vi "speed.vi"(11 "rmp":dbl) -> (3 "km/h":dbl)   [LabVIEW 2016]
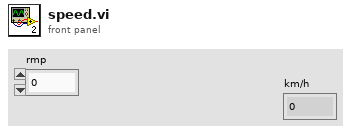
[diagram p1: front panel]
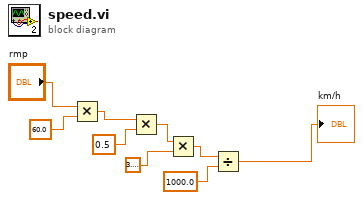
[diagram p0: block diagram]
diagram:
  n1 = Multiply(x="rmp", y=60.0) -> (x*y=w7:dbl)
  n2 = Multiply(x=w7, y=0.5) -> (x*y=w5:dbl)
  n3 = Multiply(x=w5, y=3.141592653589793) -> (x*y=w3:dbl)
  n4 = Divide(x=w3, y=1000.0) -> (x/y=→"km/h":dbl)
